vi "extract B scan data of select resolution.vi"(7 "Resolution records":i32, 9 "Data of min step":dbl[](array[numeric]), 11 "Number of records":i32) -> (3 "Array":dbl[](array[numeric]))   [LabVIEW 2014]
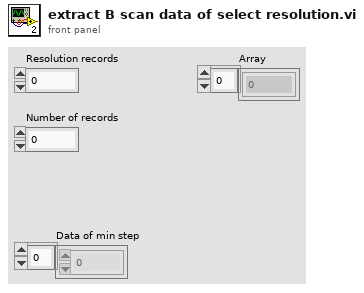
[diagram p1: front panel]
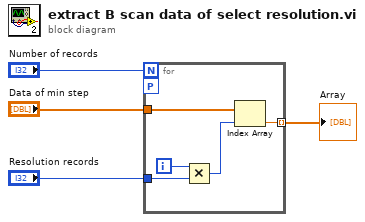
[diagram p0: block diagram]
diagram:
  n1 = for {
    N: "Number of records" -> [_]
    tunnel: [w8] -> w3 mode=indexing
    tunnel: "Data of min step" -> [w6]
    tunnel: "Resolution records" -> [w5]
    workers-P: _ -> [_]
    i -> [w7]
    n2 = Multiply(x=w7, y=w5) -> (x*y=w9:i32)
    n3 = Index Array(array=w6, index=w9) -> (element=w8:dbl)
  }
  "Array" <- w3
